vi "Convert RGB to CMYK.vi"(11 "Color in":u32(colorbox)=16777215) -> (0 "K (%)":dbl format="%#_2p", 1 "Y (%)":dbl, 2 "M (%)":dbl, 3 "C (%)":dbl)   [LabVIEW 2015, in "ColorSelector.lvclass"]
doc: "This VI will convert the RGB Color Scale to the CMYK Color Scale.\n<b> </b> <b> </b>\n©2017 Q Software Innovations, LLC (QSI)\nwritten by Quentin Alldredge\nproduced in LabVIEW 2015\n\nsupport@qsoftwareinnovations.com\nwww.qsoftwareinnovations.com\n\nAll rights reserved.\n\nRedistribution and use in source and binary forms, with or without modification, are permitted provided that the following conditions are met:\n\n * Redistributions of source code must retain the above copyright notice, this list of conditions and the following disclaimer.\n * Redistributions in binary form must reproduce the above copyright notice, this list of conditions and the following disclaimer in the documentation and/or other materials provided with the distribution.\n * Neither the name of Q Software Innovations, LLC. nor the names of its contributors may be used to endorse or promote products derived from this software without specific prior written permission.\n\nTHIS SOFTWARE IS PROVIDED BY THE COPYRIGHT HOLDERS AND CONTRIBUTORS \"AS IS\" AND ANY EXPRESS OR IMPLIED WARRANTIES, INCLUDING, BUT NOT LIMITED TO, THE IMPLIED WARRANTIES OF MERCHANTABILITY AND FITNESS FOR A PARTICULAR PURPOSE ARE DISCLAIMED. IN NO EVENT SHALL THE COPYRIGHT OWNER OR CONTRIBUTORS BE LIABLE FOR ANY DIRECT, INDIRECT, INCIDENTAL, SPECIAL, EXEMPLARY, OR CONSEQUENTIAL DAMAGES (INCLUDING, BUT NOT LIMITED TO, PROCUREMENT OF SUBSTITUTE GOODS OR SERVICES; LOSS OF USE, DATA, OR PROFITS; OR BUSINESS INTERRUPTION) HOWEVER CAUSED AND ON ANY THEORY OF LIABILITY, WHETHER IN CONTRACT, STRICT LIABILITY, OR TORT (INCLUDING NEGLIGENCE OR OTHERWISE) ARISING IN ANY WAY OUT OF THE USE OF THIS SOFTWARE, EVEN IF ADVISED OF THE POSSIBILITY OF SUCH DAMAGE."
uses:
  ColorSelector.lvclass
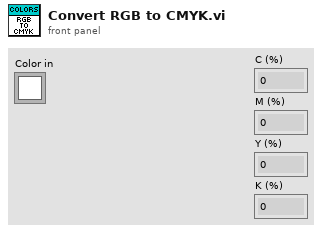
[diagram p1: front panel]
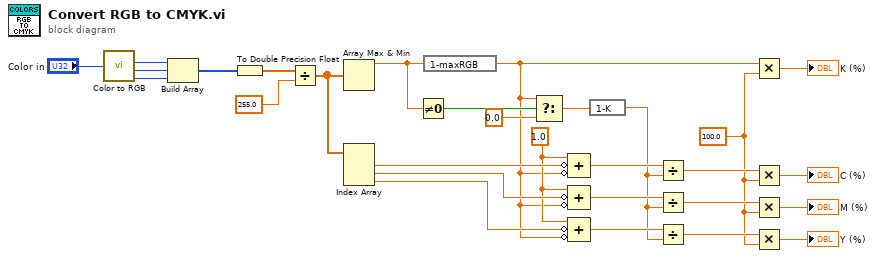
[diagram p0: block diagram]
diagram:
  w13 = 1.0
  w1 = 100.0 ("y")
  n1 = call <vilib>:"Color to RGB.vi"("Color"="Color in") -> ("R"=w24:u8, "G"=w23:u8, "B"=w22:u8)  [unwired: 1 out]
  n2 = Build Array(w24, w23, w22) -> (w28:u8[])
  n3 = To Double Precision Float(number=w28) -> (double precision float=w21:dbl[])
  n4 = Divide(x=w21, y=255.0 ("x")) -> (x/y=w20:dbl[])
  n5 = Array Max & Min(array=w20) -> (max value=w11:dbl)  [unwired: 3 out]
  n6 = Index Array(array=w20) -> (element #1=w19:dbl, element #2=w15:dbl, element #3=w12:dbl)  [unwired: 3 in]
  n7 = Not Equal To 0?(x=w11) -> (x != 0?=w10:bool)
  n8 = expression code="1-maxRGB"(w11) -> (w8:dbl)
  n9 = Select(t=w8, s=w10, f=0.0) -> (s? t:f=w7:dbl)
  n10 = Compound Arithmetic op=ADD(w13, invert w19, invert w8) -> (w18:dbl)
  n11 = Compound Arithmetic op=ADD(w13, invert w15, invert w8) -> (w16:dbl)
  n12 = Compound Arithmetic op=ADD(w13, invert w12, invert w8) -> (w14:dbl)
  n13 = expression code="1-K"(w7) -> (w6:dbl)
  n14 = Divide(x=w18, y=w6) -> (x/y=w17:dbl)
  n15 = Divide(x=w16, y=w6) -> (x/y=w4:dbl)
  n16 = Divide(x=w14, y=w6) -> (x/y=w2:dbl)
  n17 = Multiply(x=w8, y=w1) -> (x*y=→"K (%)":dbl)
  n18 = Multiply(x=w17, y=w1) -> (x*y=→"C (%)":dbl)
  n19 = Multiply(x=w4, y=w1) -> (x*y=→"M (%)":dbl)
  n20 = Multiply(x=w2, y=w1) -> (x*y=→"Y (%)":dbl)
